vi "CFTS-Menu Handler.vi"(0 "VI Refnum":refnum<vi>, 2 "Help Topic":string, 5 "Return Refnum":refnum<vi>, 7 "ItemTag":string, 11 "error in (no error)":errorcluster) -> (8 "ItemTag out":string, 15 "error out":errorcluster)   [LabVIEW 2020]
uses:
  <vilib>/printing/EasyPrintingControls.llb/layout_options.ctl
  <vilib>/printing/EasyPrintingControls.llb/orientation.ctl
  <vilib>/printing/EasyPrintingControls.llb/panel_scaling_for_page.ctl
  <vilib>/printing/EasyPrintingControls.llb/margins.ctl
  <vilib>/printing/EasyPrintingControls.llb/margin_values.ctl
  <vilib>/printing/EasyPrintingControls.llb/measurement_system.ctl
  <vilib>/printing/EasyPrintingControls.llb/printer_options.ctl
  <vilib>/printing/EasyPrintingControls.llb/printing_method.ctl
  <vilib>/printing/EasyPrintingControls.llb/color_or_monochrome.ctl
  <vilib>/printing/EasyPrintingControls.llb/page_header_options.ctl
  <vilib>/printing/EasyPrintingControls.llb/page_headers.ctl
  <vilib>/printing/EasyPrintingControls.llb/page_header_content_options.ctl
  <vilib>/printing/EasyPrintingControls.llb/contents.ctl
  <vilib>/printing/EasyPrinting.llb/Easy Print VI Panel or Documentation (refnum).vi
  <vilib>/Utility/NIReport.llb/NI_ReportGenerationCore.lvlib
panel:
  in  "layout options":T1={"orientation (unchanged)"=0, "panel scaling for page (unchanged)"=0, "margins"={"override VI margins (false)"=FALSE, "margins (1.00)"={"top"=1.0, "left"=1.0, "right"=1.0, "bottom"=1.0}, "measurement system (default)"=0}, "printer options"={"destination printer name (current)"="", "printing method (unchanged)"=0, "color or monochrome (unchanged)"=0}, "page header options"={"page headers (unchanged)"=0, "page header content options"={"Include VI Name"=TRUE, "Include VI Path"=TRUE, "Include Last Modification Date"=TRUE, "Include Date Printed"=TRUE, "Include Page Number"=TRUE, "Include VI Icon"=TRUE}}} {"page header options"."page headers (unchanged)" items=["Unchanged", "Include page headers", "Do not include page headers"]; "printer options"."color or monochrome (unchanged)" items=["Unchanged", "Color/grayscale", "Monochrome"]; "printer options"."printing method (unchanged)" items=["Unchanged", "Standard", "PostScript", "Bitmap"]; "panel scaling for page (unchanged)" items=["Unchanged", "No Scaling", "Scale front panel to fit"]; "orientation (unchanged)" items=["Unchanged", "portrait", "landscape"]; "margins"."measurement system (default)" items=["Default", "US", "Metric"]; "margins"."margins (1.00)"."right" format="%.2f"; "margins"."margins (1.00)"."bottom" format="%.2f"; "margins"."margins (1.00)"."top" format="%.2f"; "margins"."margins (1.00)"."left" format="%.2f"}
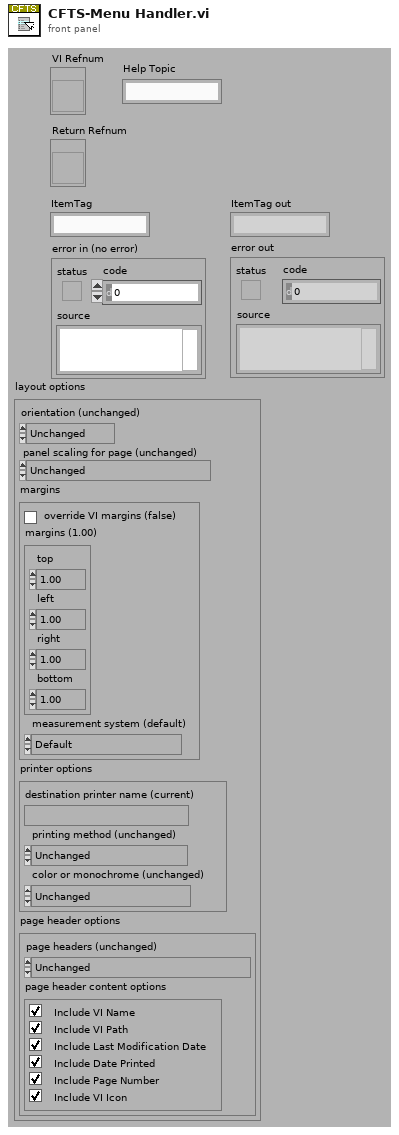
[diagram p1: front panel]
types:
  T1 = typedef "NI_ReportGenerationCore.lvlib/layout_options.ctl" = cluster{"orientation (unchanged)":T2, "panel scaling for page (unchanged)":T3, "margins":T4, "printer options":T7, "page header options":T10}
  T2 = typedef "NI_ReportGenerationCore.lvlib/orientation.ctl" = u16
  T3 = typedef "NI_ReportGenerationCore.lvlib/panel_scaling_for_page.ctl" = u16
  T4 = typedef "NI_ReportGenerationCore.lvlib/margins.ctl" = cluster{"override VI margins (false)":bool, "margins (1.00)":T5, "measurement system (default)":T6}
  T5 = typedef "NI_ReportGenerationCore.lvlib/margin_values.ctl" = cluster{"top":dbl, "left":dbl, "right":dbl, "bottom":dbl}
  T6 = typedef "NI_ReportGenerationCore.lvlib/measurement_system.ctl" = u16
  T7 = typedef "NI_ReportGenerationCore.lvlib/printer_options.ctl" = cluster{"destination printer name (current)":string, "printing method (unchanged)":T8, "color or monochrome (unchanged)":T9}
  T8 = typedef "NI_ReportGenerationCore.lvlib/printing_method.ctl" = u16
  T9 = typedef "NI_ReportGenerationCore.lvlib/color_or_monochrome.ctl" = u16
  T10 = typedef "NI_ReportGenerationCore.lvlib/page_header_options.ctl" = cluster{"page headers (unchanged)":T11, "page header content options":T12}
  T11 = typedef "NI_ReportGenerationCore.lvlib/page_headers.ctl" = u16
  T12 = typedef "NI_ReportGenerationCore.lvlib/page_header_content_options.ctl" = cluster{"Include VI Name":bool, "Include VI Path":bool, "Include Last Modification Date":bool, "Include Date Printed":bool, "Include Page Number":bool, "Include VI Icon":bool}
  T13 = typedef "NI_ReportGenerationCore.lvlib/contents.ctl" = u16
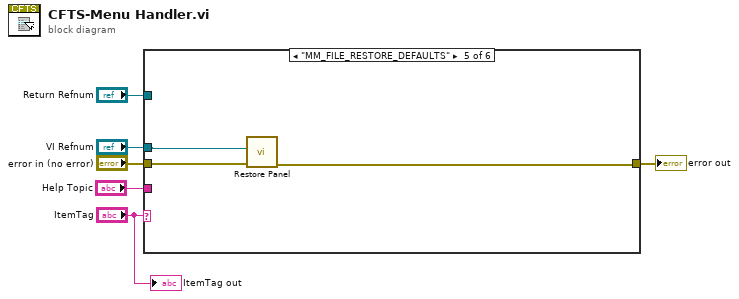
[diagram p0: block diagram]
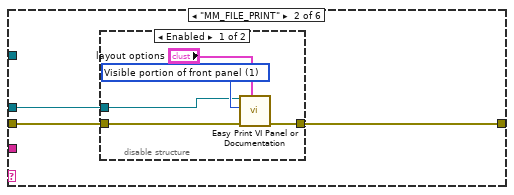
[diagram p3: hidden frame]
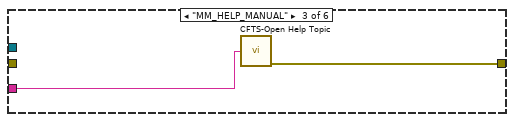
[diagram p5: hidden frame]
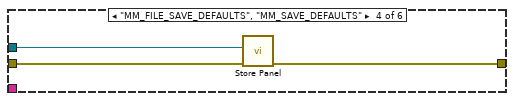
[diagram p6: hidden frame]
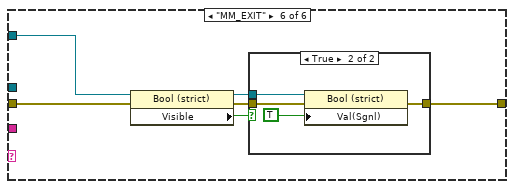
[diagram p7: hidden frame]
diagram:
  n1 = case shown="\"MM_FILE_RESTORE_DEFAULTS\"" "ItemTag" {
    tunnel: "Return Refnum" -> [_ _ _ _ _ w28]
    tunnel: "VI Refnum" -> [_ w8 _ w20 w22 _]
    tunnel: "error in (no error)" -> [w7 w10 _ w19 w23 w25]
    tunnel: [w7 w9 w17 w18 w21 w24] -> w2
    tunnel: "Help Topic" -> [_ _ w16 _ _ _]
    frame "", Default {
    }
    frame "MM_FILE_PRINT" {
      n2 = disable-structure shown="Enabled" {
        disable-tunnel: w10 -> [w14 _]
        disable-tunnel: [w13 _] -> w9
        disable-tunnel: w8 -> [w12 _]
        frame Enabled {
          w15 = T13 1 items=["Complete front panel", "Visible portion of front panel", "Icon, description, panel and diagram", "Documentation: Using the panel", "Documentation: Using as a subVI", "Documentation: Complete", "Documentation: Custom"] ("contents (complete front panel)")
          n3 = call-poly <vilib>:"Easy Print VI Panel or Documentation.vi"("layout options"="layout options", "error in (no error)"=w14, "contents (complete front panel)"=w15, "VI reference"=w12) -> ("error out"=w13:errorcluster)  [unwired: 6 in, 1 out]
        }
        frame Disabled {
        }
      }
    }
    frame "MM_HELP_MANUAL" {
      n4 = call "CFTS-Open Help Topic.vi"("Topic Keyword"=w16) -> ("error out"=w17:errorcluster)  [unwired: 14 in]
    }
    frame "MM_FILE_SAVE_DEFAULTS", "MM_SAVE_DEFAULTS" {
      n5 = call "Store Panel.vi"("error in (no error)"=w19, "VI reference"=w20) -> ("Error Out"=w18:errorcluster)  [unwired: 9 in]
    }
    frame "MM_FILE_RESTORE_DEFAULTS" {
      n6 = call "Restore Panel.vi"("Error In"=w23, "VI reference"=w22) -> ("error out"=w21:errorcluster)  [unwired: 9 in]
    }
    frame "MM_EXIT" {
      n7 = property on="Property Node" class="Bool (strict)"(reference=w28, error in=w25) -> (reference out=w27:refnum<vi>, error out=w26:errorcluster, "Visible"=w29:bool)
      n8 = case shown="True" w29 {
        tunnel: w27 -> [_ w33]
        tunnel: w26 -> [w30 w32]
        tunnel: [w30 w31] -> w24
        frame False {
        }
        frame True {
          n9 = property on="Property Node" class="Bool (strict)"(reference=w33, error in=w32, "Val(Sgnl)"=TRUE ("Value (Signaling)")) -> (error out=w31:errorcluster)  [unwired: 1 out]
        }
      }
    }
  }
  "error out" <- w2
  "ItemTag out" <- "ItemTag"
